vi "CPU_Exp_Avg_SGL.vi"(7 "exp Avg Factor":sgl, 11 "Data":sgl[](array[numeric])) -> (3 "Exp Out":sgl[](array[numeric]))   [LabVIEW 2020]
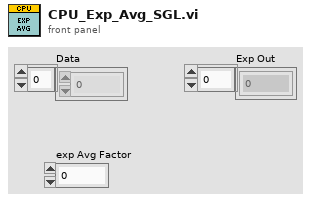
[diagram p1: front panel]
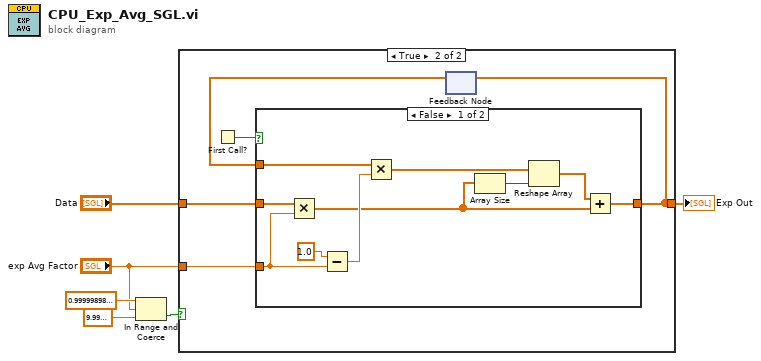
[diagram p0: block diagram]
diagram:
  n1 = In Range and Coerce(upper limit=sgl 0.999999, x="exp Avg Factor", lower limit=sgl 1e-06) -> (In Range?=w3:bool)  [unwired: 1 out]
  n2 = case shown="True" w3 {
    tunnel: "exp Avg Factor" -> [_ w12]
    tunnel: [w7 w11] -> w6
    tunnel: "Data" -> [w7 w8]
    frame False {
    }
    frame True {
      n3 = First Call?() -> (First Call?: T/F=w9:bool)
      n4 = feedback #1() -> (w10:sgl[])  [unwired: 1 in]
      n5 = case shown="False" w9 {
        tunnel: [w18 w23] -> w11
        tunnel: w10 -> [w19 _]
        tunnel: w12 -> [w16 _]
        tunnel: w8 -> [w17 w23]
        frame False {
          n6 = Multiply(x=w17, y=w16) -> (x*y=w14:sgl[])
          n7 = Subtract(x=sgl 1.0 ("y"), y=w16) -> (x-y=w21:sgl)
          n8 = Multiply(x=w19, y=w21) -> (x*y=w20:sgl[])
          n9 = Array Size(array=w14) -> (size(s)=w13:i32)
          n10 = Reshape Array(w20, w13) -> (w15:sgl[])
          n11 = Add(x=w15, y=w14) -> (x+y=w18:sgl[])
        }
        frame True {
        }
      }
      n12 = feedback-in #1(w11) -> ()
    }
  }
  "Exp Out" <- w6
